vi "Git_Add file or folder.vi"(8 "error in (no error)":errorcluster caption="entrée d'erreur (pas d'erreur)", 11 "Chemin":path) -> (0 "error out":errorcluster caption="sortie d'erreur")   [LabVIEW 2021]
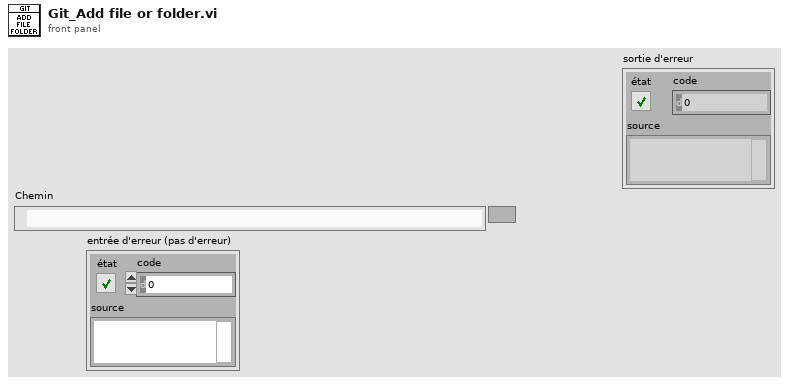
[diagram p1: front panel]
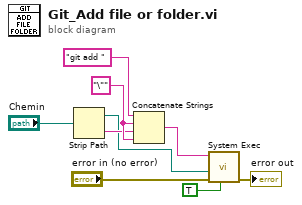
[diagram p0: block diagram]
diagram:
  w7 = "\"" ("chaîne")
  n1 = Strip Path(path="Chemin") -> (stripped path=w1:path, name=w2:string)
  n2 = Concatenate Strings("git add ", w7, w2, w7) -> (w8:string)
  n3 = call <vilib>:"System Exec.vi"("run minimized? (F)"=TRUE, "error in (no error)"="error in (no error)", "working directory"=w1, "command line"=w8) -> ("error out"=→"error out":errorcluster)  [unwired: 4 in, 3 out]
